vi "main.vi"() -> ()   [LabVIEW 2014]
panel:
  out "total steps":string
  out "map":picture
  in  "stop":bool
  in  "redo":bool
  in  "undo":bool
  in  "stage":u16(ring) items=["select stage", "1", "2", "3", "4", "5", "6", "7", "8", "9", "10"]
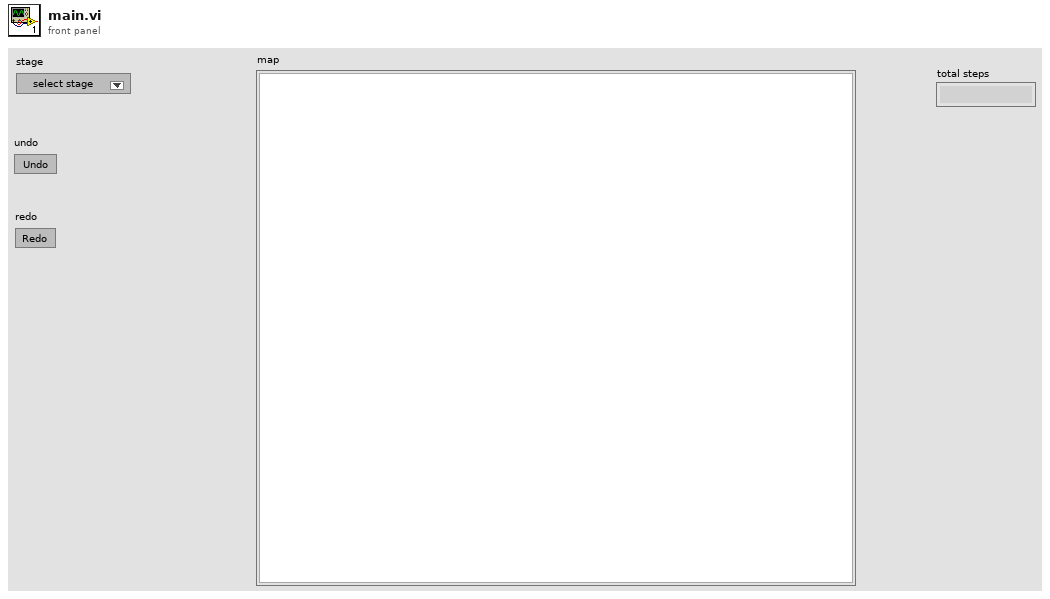
[diagram p1: front panel]
types:
  T1 = enum8{"Enabled", "Disabled", "Disabled and Grayed Out"}
  T2 = cluster{cluster{i32, i32}[], cluster{i32, i32}[], cluster{i32, i32}[], cluster{i32, i32}, i32}
  T3 = cluster{cluster{i32, i32}[], cluster{i32, i32}[], cluster{i32, i32}[], cluster{i32, i32}, i32}[]
  T4 = cluster{"Array":cluster{"Numeric":dbl, "Numeric 2":dbl}[], "Array 2":cluster{"Numeric":dbl, "Numeric 2":dbl}[], "Array 3":cluster{"Numeric":dbl, "Numeric 2":dbl}[], "Cluster":cluster{"Numeric":dbl, "Numeric 2":dbl}, "Numeric":dbl}
  T5 = cluster{"Array":cluster{"Numeric":dbl, "Numeric 2":dbl}[], "Array 2":cluster{"Numeric":dbl, "Numeric 2":dbl}[], "Array 3":cluster{"Numeric":dbl, "Numeric 2":dbl}[], "Cluster":cluster{"Numeric":dbl, "Numeric 2":dbl}, "Numeric":dbl}[]
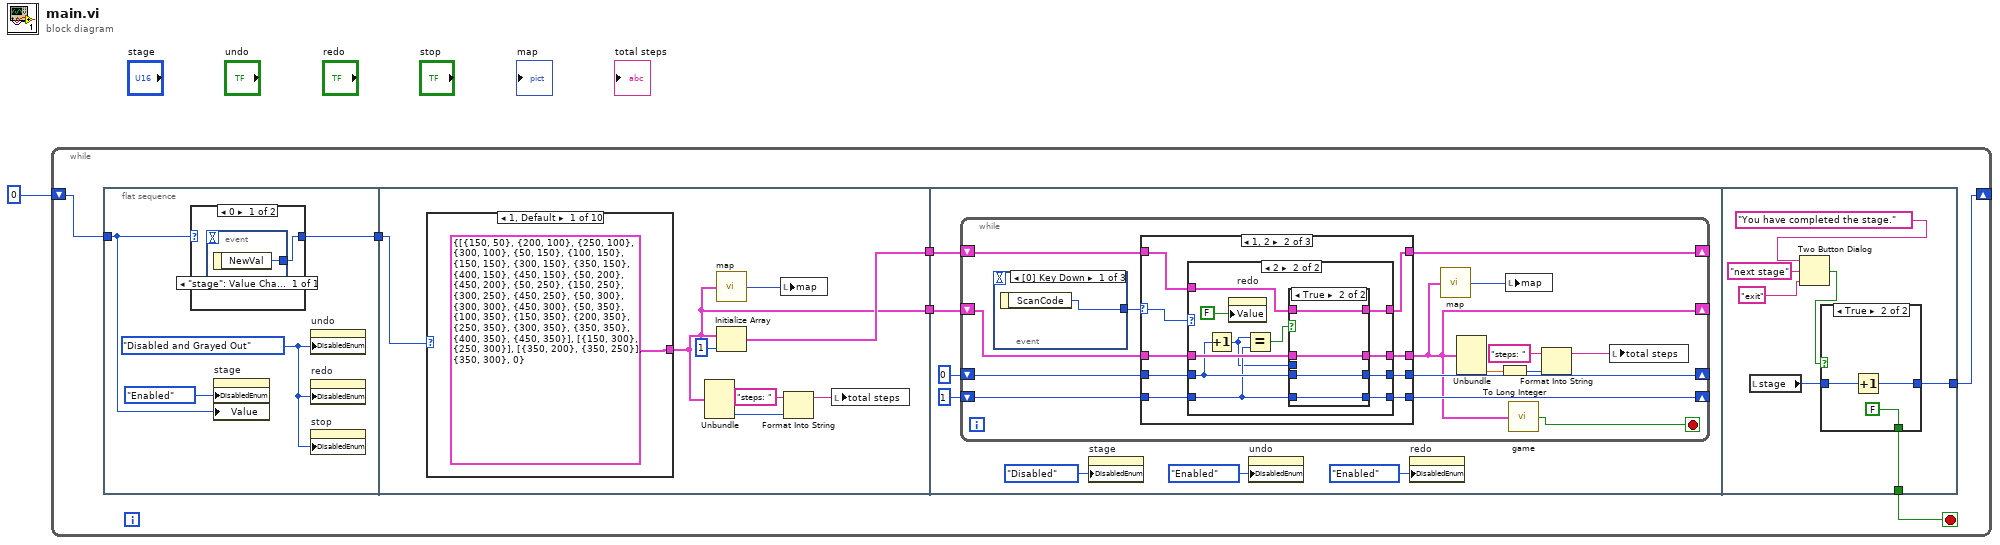
[diagram p0: block diagram]
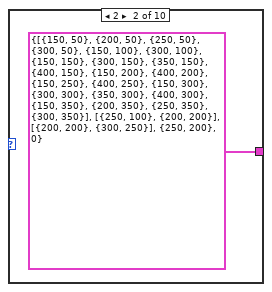
[diagram p3: hidden frame]
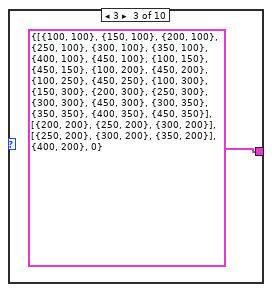
[diagram p4: hidden frame]
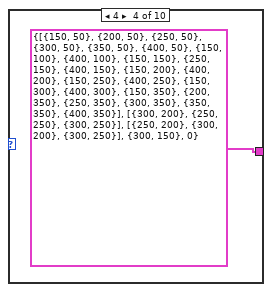
[diagram p5: hidden frame]
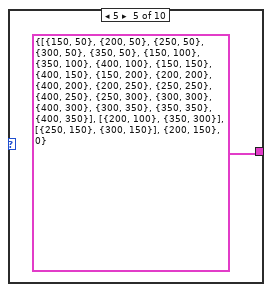
[diagram p6: hidden frame]
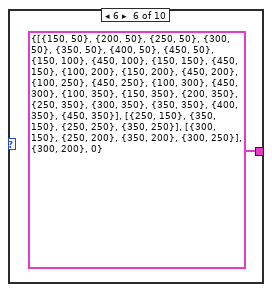
[diagram p7: hidden frame]
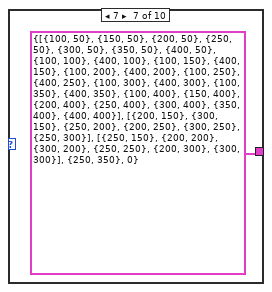
[diagram p8: hidden frame]
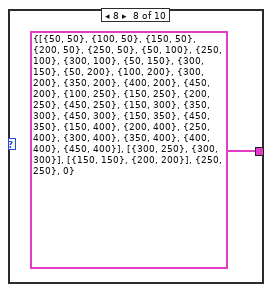
[diagram p9: hidden frame]
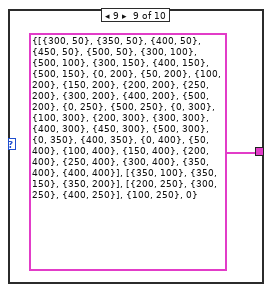
[diagram p10: hidden frame]
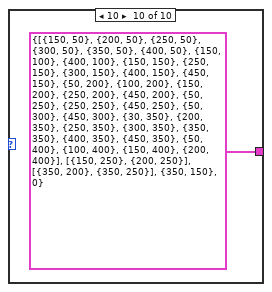
[diagram p11: hidden frame]
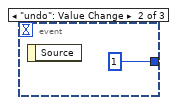
[diagram p12: hidden frame]
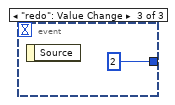
[diagram p13: hidden frame]
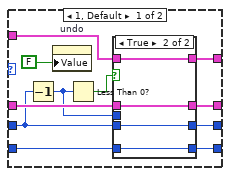
[diagram p15: hidden frame]
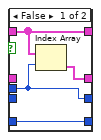
[diagram p16: hidden frame]
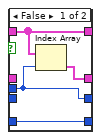
[diagram p17: hidden frame]
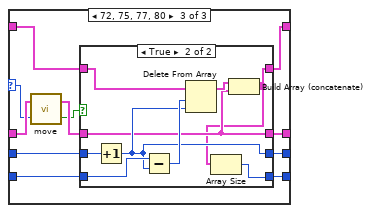
[diagram p18: hidden frame]
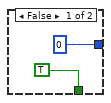
[diagram p20: hidden frame]
diagram:
  n1 = while {
    shift-right: [w3] -> _
    shift-left: 0 -> [w6]
    stop <- w2 stop-if-true
    n2 = flat-sequence {
      tunnel: [w11] -> w7
      tunnel: w6 -> [w8]
      tunnel: w7 -> [w22]
      tunnel: [w16] -> w5
      tunnel: [w15] -> w4
      tunnel: w5 -> [w39]
      tunnel: w4 -> [w38]
      tunnel: [w134] -> w3
      tunnel: [w133] -> w2
      frame #0 {
        w10 = T1."Disabled and Grayed Out" ("Disabled")
        n3 = case shown="0" w8 {
          selector: w8 -> [_ w14]
          tunnel: [w12 w14] -> w11
          frame 0 {
            n4 = event shown="[0] \"stage\": Value Change" {
              selector: _ -> [_]
              dyn-events: _ -> [_]
              timeout: _ -> [_]
              tunnel: [w13] -> w12
              event "stage": Value Change {
                n5 = event-data() -> ("NewVal"=w13:u16)  [unwired: 1 in]
              }
            }
          }
          frame 1, Default {
          }
        }
        n6 = property on="stage" class="Ring (strict)"("DisabledEnum"=T1."Enabled" ("Disabled"), "Value"=w8) -> ()  [unwired: 2 in, 2 out]
        n7 = property on="undo" class="Bool (strict)"("DisabledEnum"=w10) -> ()  [unwired: 2 in, 2 out]
        n8 = property on="redo" class="Bool (strict)"("DisabledEnum"=w10) -> ()  [unwired: 2 in, 2 out]
        n9 = property on="stop" class="Bool (strict)"("DisabledEnum"=w10) -> ()  [unwired: 2 in, 2 out]
      }
      frame #1 {
        n10 = case shown="1, Default" w22 {
          tunnel: [T2 {[{150, 50}, {200, 100}, {250, 100}, {300, 100}, {50, 150}, {100, 150}, {150, 150}, {300, 150}, {350, 150}, {400, 150}, {450, 150}, {50, 200}, {450, 200}, {50, 250}, {150, 250}, {300, 250}, {450, 250}, {50, 300}, {300, 300}, {450, 300}, {50, 350}, {100, 350}, {150, 350}, {200, 350}, {250, 350}, {300, 350}, {350, 350}, {400, 350}, {450, 350}], [{150, 300}, {250, 300}], [{350, 200}, {350, 250}], {350, 300}, 0} T2 {[{150, 50}, {200, 50}, {250, 50}, {300, 50}, {150, 100}, {300, 100}, {150, 150}, {300, 150}, {350, 150}, {400, 150}, {150, 200}, {400, 200}, {150, 250}, {400, 250}, {150, 300}, {300, 300}, {350, 300}, {400, 300}, {150, 350}, {200, 350}, {250, 350}, {300, 350}], [{250, 100}, {200, 200}], [{200, 200}, {300, 250}], {250, 200}, 0} T2 {[{100, 100}, {150, 100}, {200, 100}, {250, 100}, {300, 100}, {350, 100}, {400, 100}, {450, 100}, {100, 150}, {450, 150}, {100, 200}, {450, 200}, {100, 250}, {450, 250}, {100, 300}, {150, 300}, {200, 300}, {250, 300}, {300, 300}, {450, 300}, {300, 350}, {350, 350}, {400, 350}, {450, 350}], [{200, 200}, {250, 200}, {300, 200}], [{250, 200}, {300, 200}, {350, 200}], {400, 200}, 0} T2 {[{150, 50}, {200, 50}, {250, 50}, {300, 50}, {350, 50}, {400, 50}, {150, 100}, {400, 100}, {150, 150}, {250, 150}, {400, 150}, {150, 200}, {400, 200}, {150, 250}, {400, 250}, {150, 300}, {400, 300}, {150, 350}, {200, 350}, {250, 350}, {300, 350}, {350, 350}, {400, 350}], [{300, 200}, {250, 250}, {300, 250}], [{250, 200}, {300, 200}, {300, 250}], {300, 150}, 0} T2 {[{150, 50}, {200, 50}, {250, 50}, {300, 50}, {350, 50}, {150, 100}, {350, 100}, {400, 100}, {150, 150}, {400, 150}, {150, 200}, {200, 200}, {400, 200}, {200, 250}, {250, 250}, {400, 250}, {250, 300}, {300, 300}, {400, 300}, {300, 350}, {350, 350}, {400, 350}], [{200, 100}, {350, 300}], [{250, 150}, {300, 150}], {200, 150}, 0} T2 {[{150, 50}, {200, 50}, {250, 50}, {300, 50}, {350, 50}, {400, 50}, {450, 50}, {150, 100}, {450, 100}, {150, 150}, {450, 150}, {100, 200}, {150, 200}, {450, 200}, {100, 250}, {450, 250}, {100, 300}, {450, 300}, {100, 350}, {150, 350}, {200, 350}, {250, 350}, {300, 350}, {350, 350}, {400, 350}, {450, 350}], [{250, 150}, {350, 150}, {250, 250}, {350, 250}], [{300, 150}, {250, 200}, {350, 200}, {300, 250}], {300, 200}, 0} T2 {[{100, 50}, {150, 50}, {200, 50}, {250, 50}, {300, 50}, {350, 50}, {400, 50}, {100, 100}, {400, 100}, {100, 150}, {400, 150}, {100, 200}, {400, 200}, {100, 250}, {400, 250}, {100, 300}, {400, 300}, {100, 350}, {400, 350}, {100, 400}, {150, 400}, {200, 400}, {250, 400}, {300, 400}, {350, 400}, {400, 400}], [{200, 150}, {300, 150}, {250, 200}, {200, 250}, {300, 250}, {250, 300}], [{250, 150}, {200, 200}, {300, 200}, {250, 250}, {200, 300}, {300, 300}], {250, 350}, 0} T2 {[{50, 50}, {100, 50}, {150, 50}, {200, 50}, {250, 50}, {50, 100}, {250, 100}, {300, 100}, {50, 150}, {300, 150}, {50, 200}, {100, 200}, {300, 200}, {350, 200}, {400, 200}, {450, 200}, {100, 250}, {150, 250}, {200, 250}, {450, 250}, {150, 300}, {350, 300}, {450, 300}, {150, 350}, {450, 350}, {150, 400}, {200, 400}, {250, 400}, {300, 400}, {350, 400}, {400, 400}, {450, 400}], [{300, 250}, {300, 300}], [{150, 150}, {200, 200}], {250, 250}, 0} T2 {[{300, 50}, {350, 50}, {400, 50}, {450, 50}, {500, 50}, {300, 100}, {500, 100}, {300, 150}, {400, 150}, {500, 150}, {0, 200}, {50, 200}, {100, 200}, {150, 200}, {200, 200}, {250, 200}, {300, 200}, {400, 200}, {500, 200}, {0, 250}, {500, 250}, {0, 300}, {100, 300}, {200, 300}, {300, 300}, {400, 300}, {450, 300}, {500, 300}, {0, 350}, {400, 350}, {0, 400}, {50, 400}, {100, 400}, {150, 400}, {200, 400}, {250, 400}, {300, 400}, {350, 400}, {400, 400}], [{350, 100}, {350, 150}, {350, 200}], [{200, 250}, {300, 250}, {400, 250}], {100, 250}, 0} T2 {[{150, 50}, {200, 50}, {250, 50}, {300, 50}, {350, 50}, {400, 50}, {150, 100}, {400, 100}, {150, 150}, {250, 150}, {300, 150}, {400, 150}, {450, 150}, {50, 200}, {100, 200}, {150, 200}, {250, 200}, {450, 200}, {50, 250}, {250, 250}, {450, 250}, {50, 300}, {450, 300}, {30, 350}, {200, 350}, {250, 350}, {300, 350}, {350, 350}, {400, 350}, {450, 350}, {50, 400}, {100, 400}, {150, 400}, {200, 400}], [{150, 250}, {200, 250}], [{350, 200}, {350, 250}], {350, 150}, 0}] -> w15
          frame 1, Default {
          }
          frame 2 {
          }
          frame 3 {
          }
          frame 4 {
          }
          frame 5 {
          }
          frame 6 {
          }
          frame 7 {
          }
          frame 8 {
          }
          frame 9 {
          }
          frame 10 {
          }
        }
        n11 = Unbundle(w15) -> (w19:i32)  [unwired: 4 out]
        n12 = call "map.vi"("Cluster 2"=w15) -> ("new picture"=w20:picture)
        n13 = Initialize Array(w15, 1 ("dimension size")) -> (w16:T3)
        n14 = local write "map"(w20) -> ()
        n15 = Format Into String(initial string="steps: ", w19) -> (resulting string=w17:string)  [unwired: 2 in, 1 out]
        n16 = local write "total steps"(w17) -> ()
      }
      frame #2 {
        n17 = while {
          shift-right: [w52] -> _
          shift-left: w39 -> [w53]
          shift-right: [w43] -> _
          shift-left: w38 -> [w51]
          shift-right: [w48] -> _
          shift-left: 0 -> [w50]
          shift-right: [w47] -> _
          shift-left: 1 -> [w49]
          stop <- w42 stop-if-true
          n18 = event shown="[0] Key Down" {
            selector: _ -> [_ _ _]
            dyn-events: _ -> [_ _ _]
            timeout: _ -> [_ _ _]
            tunnel: [w55 1 2] -> w54
            event Key Down {
              n19 = event-data() -> ("ScanCode"=w55:i16)  [unwired: 1 in]
            }
            event "undo": Value Change {
              n20 = event-data() -> ()  [unwired: 1 in, 1 out]
            }
            event "redo": Value Change {
              n21 = event-data() -> ()  [unwired: 1 in, 1 out]
            }
          }
          n22 = case shown="1, 2" w54 {
            selector: w54 -> [_ w70 w110]
            tunnel: w53 -> [w61 w69 w119]
            tunnel: [w61 w68 w118] -> w52
            tunnel: w51 -> [w60 w66 w112]
            tunnel: [w60 w67 w117] -> w43
            tunnel: w50 -> [w59 w65 w116]
            tunnel: w49 -> [w58 w63 w114]
            tunnel: [w59 w64 w115] -> w48
            tunnel: [w58 w62 w113] -> w47
            frame 0, Default {
            }
            frame 1, 2 {
              n23 = case shown="2" w70 {
                tunnel: w69 -> [w79 w99]
                tunnel: [w78 w98] -> w68
                tunnel: [w77 w97] -> w67
                tunnel: w66 -> [w76 w96]
                tunnel: w65 -> [w72 w93]
                tunnel: [w75 w95] -> w64
                tunnel: w63 -> [w74 w91]
                tunnel: [w73 w94] -> w62
                frame 1, Default {
                  n24 = Decrement(x=w72) -> (x-1=w71:i32)
                  n25 = property on="undo" class="Bool (strict)"("Value"=FALSE) -> ()  [unwired: 2 in, 2 out]
                  n26 = Less Than 0?(x=w71) -> (x < 0?=w81:bool)
                  n27 = case shown="True" w81 {
                    tunnel: w79 -> [w85 w89]
                    tunnel: [w85 w89] -> w78
                    tunnel: [w84 w88] -> w77
                    tunnel: w76 -> [_ w88]
                    tunnel: w72 -> [_ w87]
                    tunnel: [w83 w87] -> w75
                    tunnel: w74 -> [w82 w86]
                    tunnel: [w82 w86] -> w73
                    tunnel: w71 -> [w83 _]
                    frame False {
                      n28 = Index Array(array=w85, index=w83) -> (element=w84:T4)
                    }
                    frame True {
                    }
                  }
                }
                frame 2 {
                  n29 = Increment(x=w93) -> (x+1=w90:i32)
                  n30 = property on="redo" class="Bool (strict)"("Value"=FALSE) -> ()  [unwired: 2 in, 2 out]
                  n31 = Equal?(x=w90, y=w91) -> (x = y?=w100:bool)
                  n32 = case shown="True" w100 {
                    tunnel: w99 -> [w104 w108]
                    tunnel: [w104 w108] -> w98
                    tunnel: [w103 w107] -> w97
                    tunnel: w96 -> [_ w107]
                    tunnel: w93 -> [_ w106]
                    tunnel: [w101 w106] -> w95
                    tunnel: w91 -> [w102 w105]
                    tunnel: [w102 w105] -> w94
                    tunnel: w90 -> [w101 _]
                    frame False {
                      n33 = Index Array(array=w104, index=w101) -> (element=w103:T4)
                    }
                    frame True {
                    }
                  }
                }
              }
            }
            frame 72, 75, 77, 80 {
              n34 = call "move.vi"("Numeric"=w110, "Cluster 2"=w112) -> ("Boolean"=w109:bool, "Cluster 3"=w111:T4)
              n35 = case shown="True" w109 {
                tunnel: w119 -> [w123 w124]
                tunnel: [w123 w125] -> w118
                tunnel: w111 -> [w122 w127]
                tunnel: [w122 w127] -> w117
                tunnel: w116 -> [w121 w132]
                tunnel: [w121 w129] -> w115
                tunnel: w114 -> [w120 w131]
                tunnel: [w120 w126] -> w113
                frame False {
                }
                frame True {
                  n36 = Increment(x=w132) -> (x+1=w129:i32)
                  n37 = Subtract(x=w131, y=w129) -> (x-y=w130:i32)
                  n38 = Delete From Array(array=w124, length=w130, index=w129) -> (array with subset deleted=w128:T5)  [unwired: 1 out]
                  n39 = Build Array (concatenate)(w128, w127) -> (w125:T5)
                  n40 = Array Size(array=w125) -> (size(s)=w126:i32)
                }
              }
            }
          }
          n41 = call "map.vi"("Cluster 2"=w43) -> ("new picture"=w46:picture)
          n42 = Unbundle(w43) -> ("Numeric"=w41:dbl)  [unwired: 4 out]
          n43 = To Long Integer(number=w41) -> (32bit integer=w40:i32)
          n44 = local write "map"(w46) -> ()
          n45 = call "game.vi"("Cluster 2"=w43) -> ("x = y?"=w42:bool)
          n46 = Format Into String(initial string="steps: ", w40) -> (resulting string=w44:string)  [unwired: 2 in, 1 out]
          n47 = local write "total steps"(w44) -> ()
        }
        n48 = property on="stage" class="Ring (strict)"("DisabledEnum"=T1."Disabled" ("Disabled")) -> ()  [unwired: 2 in, 2 out]
        n49 = property on="undo" class="Bool (strict)"("DisabledEnum"=T1."Enabled" ("Disabled")) -> ()  [unwired: 2 in, 2 out]
        n50 = property on="redo" class="Bool (strict)"("DisabledEnum"=T1."Enabled" ("Disabled")) -> ()  [unwired: 2 in, 2 out]
      }
      frame #3 {
        n51 = local read "stage"() -> (w135:u16)
        n52 = Two Button Dialog(message="You have completed the stage.", 1:"exit" ("F button name (\"Cancel\")"), 2:"next stage" ("T button name (\"OK\")")) -> (T button?=w136:bool)
        n53 = case shown="True" w136 {
          tunnel: w135 -> [_ w144]
          tunnel: [0 w143] -> w134
          tunnel: [TRUE FALSE] -> w133
          frame False {
          }
          frame True {
            n54 = Increment(x=w144) -> (x+1=w143:u16)
          }
        }
      }
    }
  }
